vi "Test Failing.vi"() -> ()   [LabVIEW 2020, in "Failing Test Case.lvclass"]
doc: "Failing test"
uses:
  Failing Test Case.lvclass
  Passing Test Case/Passing Test Case.lvclass
  C:/git/astemes-lunit/source/Framework/Test Case/LUnit Test Case.lvclass
  Framework/Test Case/LUnit Test Case.lvclass/LUnit Test Case.ctl
  Framework/Test Case/Assertions/Fail.vi
  Framework/Test Case/Assertions/Pass.vi
  Framework/Test Case/Private/SubVIs/Set Assertion Type.vi
  Framework/Test Case/Private/SubVIs/Add test result.vi
  Framework/Result Types/Case Result/Public/Record Assertion Result.vi
  Framework/Result Types/Method Result/Public/Aggregate Assertion Results.vi
  Framework/Result Types/Method Result/Private/Merge Status.vi
  Framework/Result Types/Method Result/Private/Concatenate result strings.vi
  Framework/Test Case/LUnit Test Case.lvclass
panel:
  out "Passing Test Case Out":refnum<class "Passing Test Case.lvclass">
  in  "Passing Test Case In":refnum<class "Passing Test Case.lvclass">
  out "error out":errorcluster
  in  "error in (no error)":errorcluster
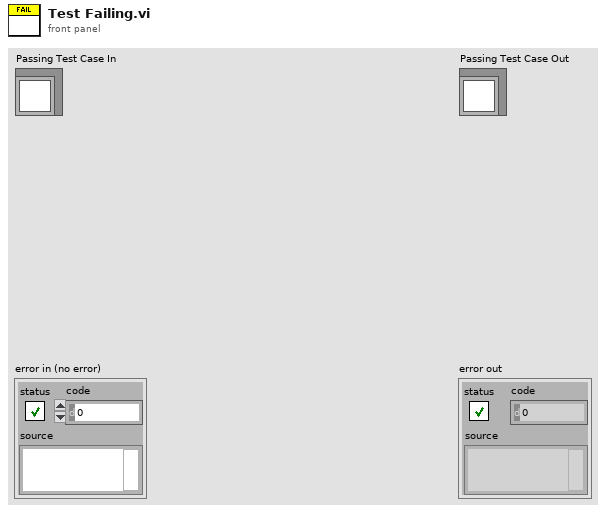
[diagram p1: front panel]
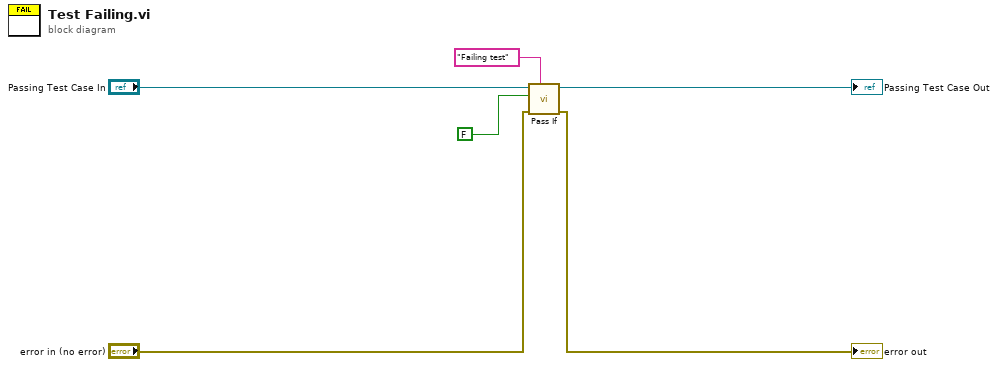
[diagram p0: block diagram]
diagram:
  n1 = call "Pass If.vi"("Description"="Failing test", "error in (no error)"="error in (no error)", "Pass?"=FALSE, "LUnit Test Case In"="Passing Test Case In") -> ("error out"=→"error out":errorcluster, "LUnit Test Case Out"=→"Passing Test Case Out":refnum<class "Passing Test Case.lvclass">)  [unwired: 6 in]
